vi "Initialize Settings.vi"(8 "error in (no error)":errorcluster, 10 "thread settings":T1, 11 "PXImc Transceiver in":refnum<class "DSF PXImc Transceiver.lvclass">) -> (0 "error out":errorcluster, 3 "PXImc Transceiver out":refnum<class "DSF PXImc Transceiver.lvclass">)   [LabVIEW 2017, in "DSF Core.lvlib" / "DSF PXImc Transceiver.lvclass"]
uses:
  DSF PXImc Transceiver.lvclass
  Typedefs/DSF Settings Info.ctl
  DSF PXImc Transceiver.lvclass/DSF PXImc Transceiver.ctl
  Bad Setting Error.vi
  Classes/Configuration/Configuration Session.lvclass
  DSF Core.lvlib
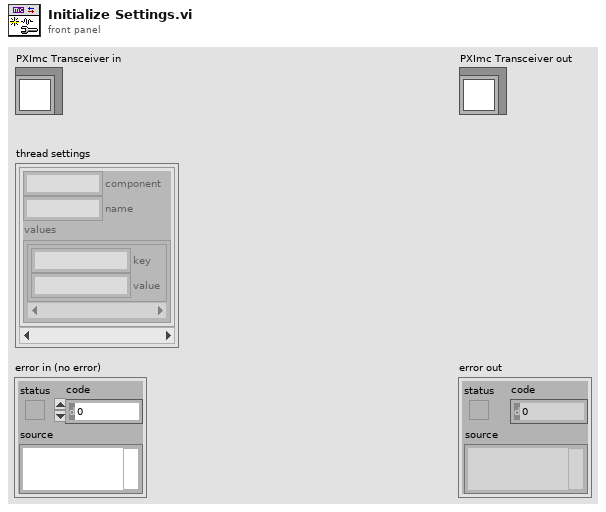
[diagram p1: front panel]
types:
  T1 = typedef "DSF Core.lvlib/DSF Settings Info.ctl" = cluster{"component":string, "name":string, "values":cluster{"key":string, "value":string}[]}[]
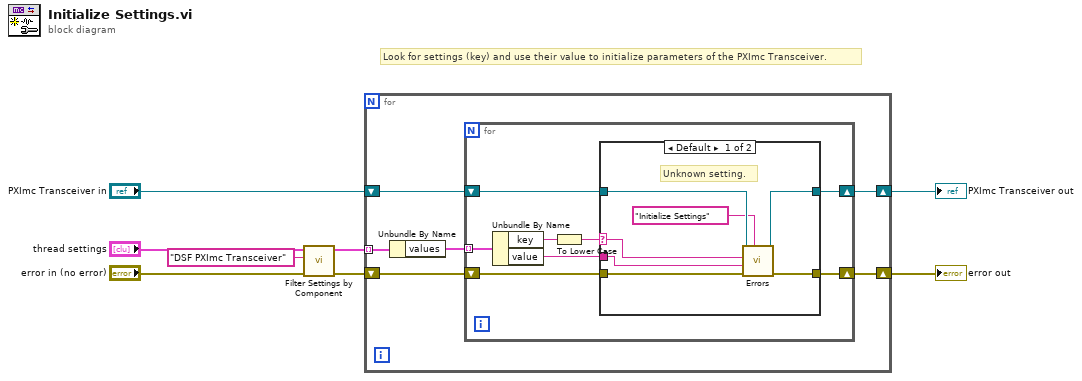
[diagram p0: block diagram]
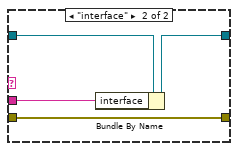
[diagram p2: hidden frame]
diagram:
  # "Look for settings (key) and use their value to initialize parameters of the PXImc Transceiver."
  n1 = call "Filter Settings by Component.vi"("error in (no error)"="error in (no error)", "component"="DSF PXImc Transceiver", "settings"="thread settings") -> ("error out"=w5:errorcluster, "filtered settings"=w3:T1)  [unwired: 7 in]
  n2 = for {
    shift-right: [w13] -> w4
    shift-left: w5 -> [w14]
    tunnel: w3 -> [w12] mode=indexing
    shift-right: [w9] -> w1
    shift-left: "PXImc Transceiver in" -> [w10]
    n3 = Unbundle By Name(w12) -> ("values"=w11:cluster{"key":string, "value":string}[])
    n4 = for {
      shift-right: [w18] -> w13
      shift-left: w14 -> [w21]
      tunnel: w11 -> [w22] mode=indexing
      shift-right: [w15] -> w9
      shift-left: w10 -> [w16]
      n5 = Unbundle By Name(w22) -> ("key"=w20:string, "value"=w19:string)
      n6 = To Lower Case(string=w20) -> (all lower case string=w17:string)
      n7 = case shown="Default" w17 {
        selector: w17 -> [w23 _]
        tunnel: w21 -> [w29 w32]
        tunnel: w19 -> [w24 w31]
        tunnel: [w28 w32] -> w18
        tunnel: w16 -> [w27 w33]
        tunnel: [w26 w30] -> w15
        frame Default {
          # "Unknown setting."
          n8 = call-poly "Errors.vi"("vi name"="Initialize Settings", "error in (no error)"=w29, "value"=w24, "key"=w23, "PXImc Transceiver in"=w27) -> ("error out"=w28:errorcluster, "PXImc Transceiver out"=w26:refnum<class "DSF PXImc Transceiver.lvclass">)  [unwired: 5 in]
        }
        frame "interface" {
          n9 = Bundle By Name(cluster=w33, "interface"=w31) -> (w30:refnum<class "DSF PXImc Transceiver.lvclass">)
        }
      }
    }
  }
  "error out" <- w4
  "PXImc Transceiver out" <- w1
